vi "Configure Export Signal.vi"(8 "error in":errorcluster, 11 "FGen PXI Base CFG in":refnum<class "Generate DC CFG.lvclass">) -> (0 "error out":errorcluster, 3 "FGen PXI Base CFG out":refnum<class "Generate DC CFG.lvclass">)   [LabVIEW 2023, in "FGen Simulated CFGs.lvlib" / "Generate DC CFG.lvclass"]
uses:
  Generate DC CFG.lvclass
  Configuration/Configuration JSON/Configuration JSON Base/CFG JSON.lvclass/CFG JSON.ctl
  83dfbe61-3606-4481-8714-31fd42503d22.vi
  <vilib>/JDP Science/JSONtext/Find Item.vi
  <vilib>/JDP Science/JSONtext/Next JSON Value.vi
  <vilib>/JDP Science/JSONtext/String Subset.vi
  <vilib>/JDP Science/JSONtext/Parsing/Advance past next JSON Value (inlined COPY).vi
  <vilib>/JDP Science/JSONtext/Parsing/Advance past whitespace.vi
  <vilib>/JDP Science/JSONtext/Parsing/Advance past String.vi
  <vilib>/JDP Science/JSONtext/Parsing/Advance past Number.vi
  <vilib>/JDP Science/JSONtext/Parsing/Advance past Line Ending.vi
  <vilib>/JDP Science/JSONtext/Parsing/Parse Full Path or Item Name.vi
  <vilib>/JDP Science/JSONtext/Parsing/Advance past Array.vi
  <vilib>/JDP Science/JSONtext/Parsing/Advance past Object.vi
  <vilib>/JDP Science/JSONtext/support/Error Cluster From Code.vi
  <vilib>/JDP Science/JSONtext/Offset/Find Item Locations by Path.vi
  <vilib>/JDP Science/JSONtext/JSON text to Variant.vi
  <vilib>/Utility/error.llb/Error Cluster From Error Code.vi
  <vilib>/JDP Science/JSONtext/LVClass Serializer/JSONtext LVClass Serializer.lvclass
  <vilib>/ErrorRing/Error Ring.xnode
  Generate DC CFG.lvclass/Generate DC CFG.ctl
  Configuration/Configuration JSON/Configuration JSON Base/CFG JSON.lvclass
  D:/git/HAL/HAL GOOP4/Configuration/Configuration JSON/Configuration JSON Base/CFG JSON.lvclass
  D:/git/HAL/HAL GOOP4/Interfaces/IConfigure/IConfigure.lvclass
  D:/git/HAL/HAL GOOP4/FGen/FGen Simulated/Configurations/Generate DC CFG/Generate DC CFG.lvclass
panel:
  out "Data":T1
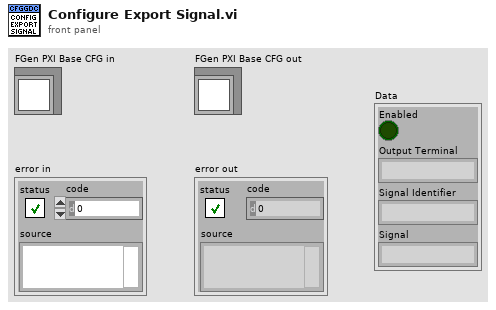
[diagram p1: front panel]
types:
  T1 = cluster{"Enabled":bool, "Output Terminal":string, "Signal Identifier":string, "Signal":string}
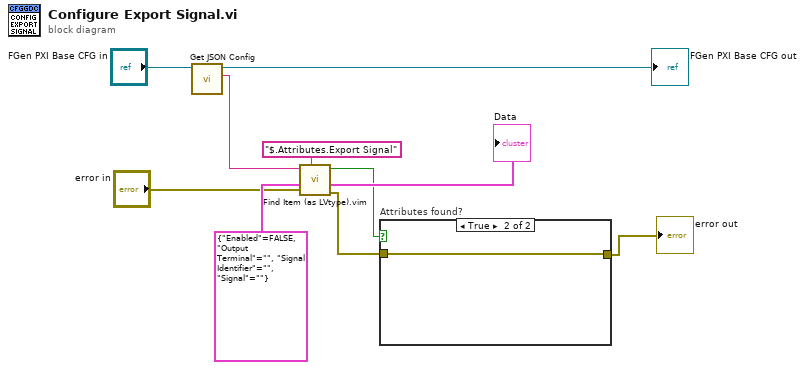
[diagram p0: block diagram]
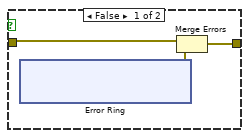
[diagram p2: hidden frame]
diagram:
  n1 = call "Get JSON Config.vi"("CFG Base in"="FGen PXI Base CFG in") -> ("<JSON>Config>"=w6:string, "CFG Base out"=→"FGen PXI Base CFG out":refnum<class "Generate DC CFG.lvclass">)  [unwired: 9 in]
  n2 = call "Find Item (as LVtype).vim"("$Path or Item Name"="$.Attributes.Export Signal", "error in (no error)"="error in", "Data Type and Default Value"=T1 {"Enabled"=FALSE, "Output Terminal"="", "Signal Identifier"="", "Signal"=""}, "JSON"=w6) -> ("error out"=w4:errorcluster, "Data"=→"Data":T1, "Found"=w3:bool)  [unwired: 4 in, 1 out]
  n3 = case "Attributes found?" shown="True" w3 {
    tunnel: [w13 w19] -> w2
    tunnel: w4 -> [w12 w19]
    frame False {
      n4 = xnode "Error Ring"() -> ("error out"=w11:errorcluster)
      n5 = Merge Errors(w12, w11) -> (w13:errorcluster)
    }
    frame True {
    }
  }
  "error out" <- w2
